vi "Parse Semver Range.vi"(8 "error in (no error)":errorcluster, 9 "Offset in":i32, 10 "Range Specifier":string) -> (0 "error out":errorcluster, 1 "Offset out":i32, 2 "Operator":string, 3 "Semver out":refnum<class "Semver.lvclass">)   [LabVIEW 2017, in "Semver.lvlib" / "Semver.lvclass"]
uses:
  Semver.lvclass
  Semver.lvclass/Semver.ctl
  <vilib>/Utility/error.llb/Error Cluster From Error Code.vi
  <vilib>/ErrorRing/Error Ring.xnode
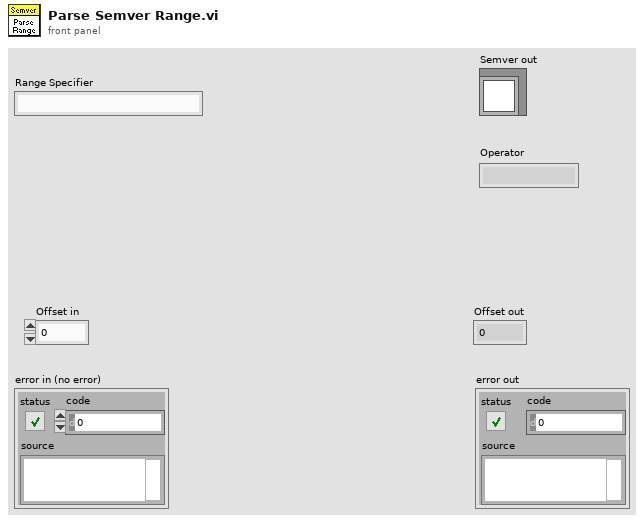
[diagram p1: front panel]
types:
  T1 = enum16{"Strip Chars", "Find Major", "Find Minor", "Find Patch", "Find Pre-Release", "Find Meta-Data"}
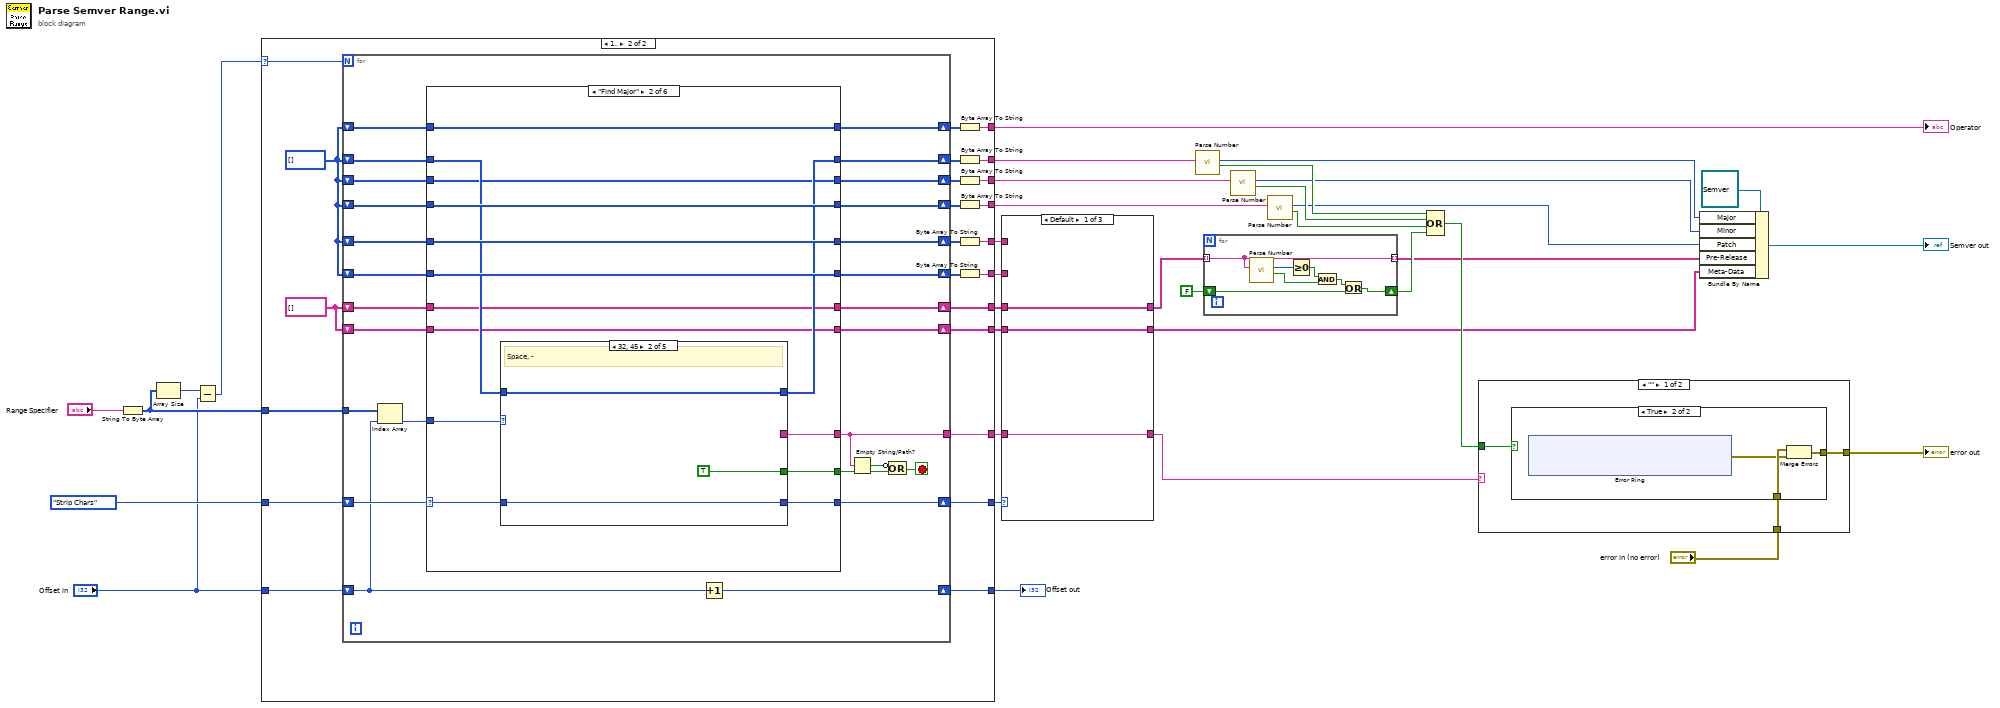
[diagram p0: block diagram]
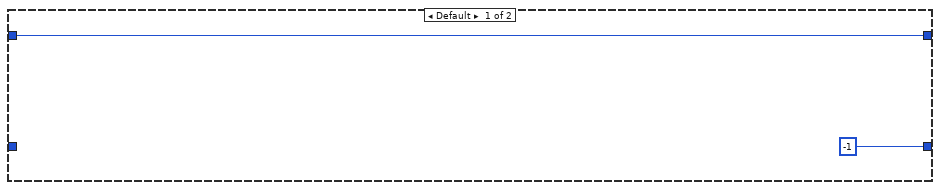
[diagram p2: hidden frame]
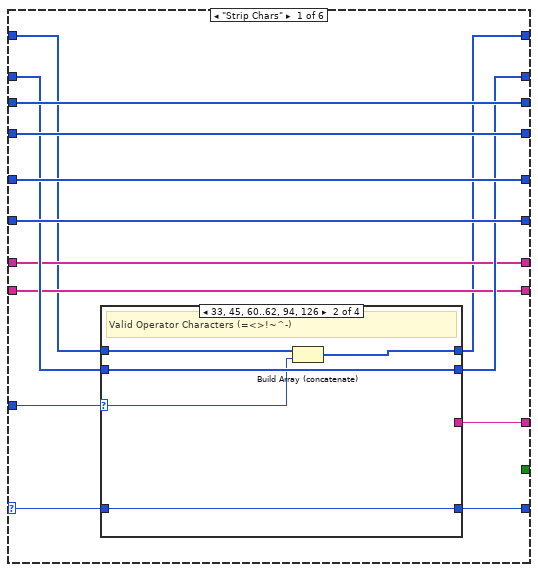
[diagram p3: hidden frame]
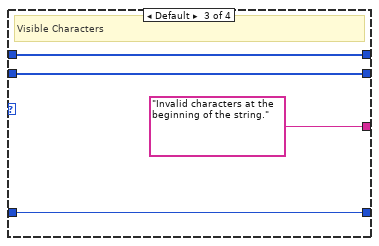
[diagram p5: hidden frame]
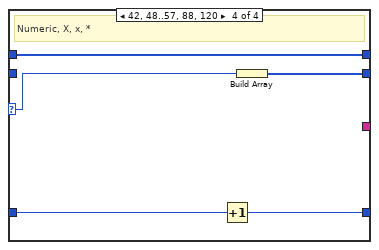
[diagram p6: hidden frame]
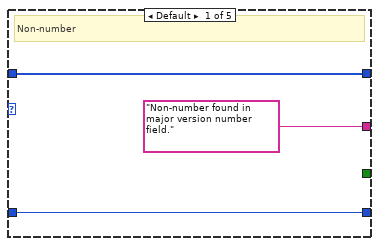
[diagram p7: hidden frame]
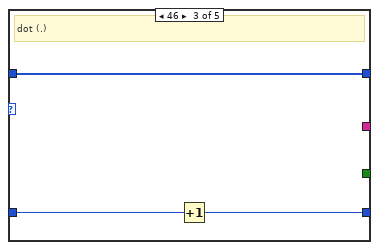
[diagram p8: hidden frame]
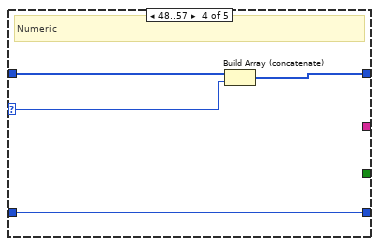
[diagram p9: hidden frame]
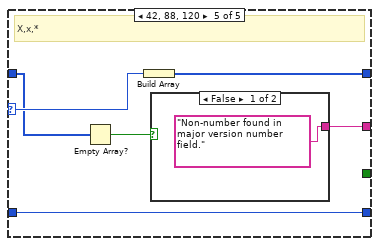
[diagram p10: hidden frame]
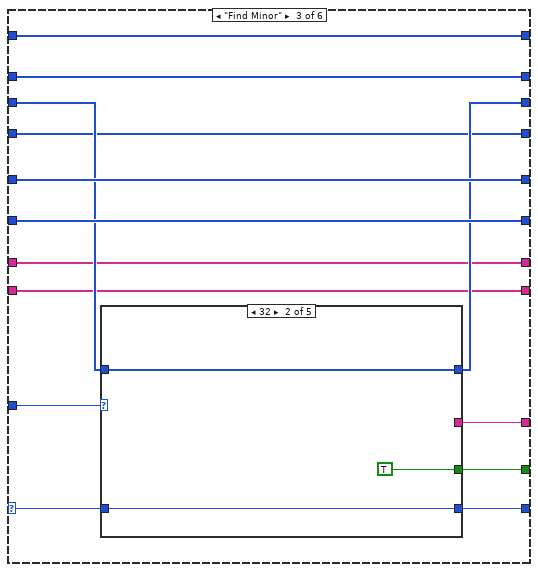
[diagram p12: hidden frame]
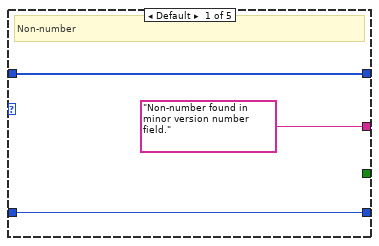
[diagram p13: hidden frame]
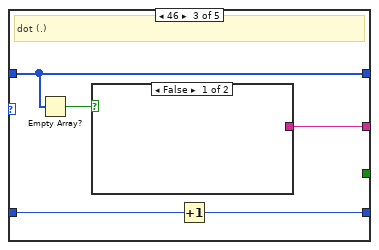
[diagram p14: hidden frame]
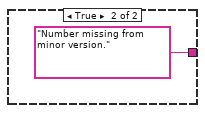
[diagram p15: hidden frame]
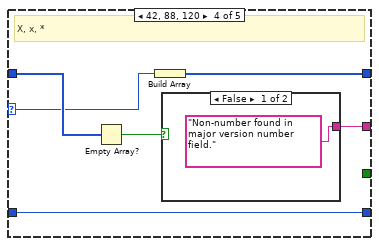
[diagram p16: hidden frame]
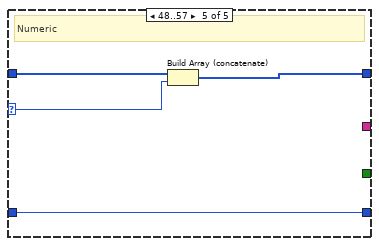
[diagram p18: hidden frame]
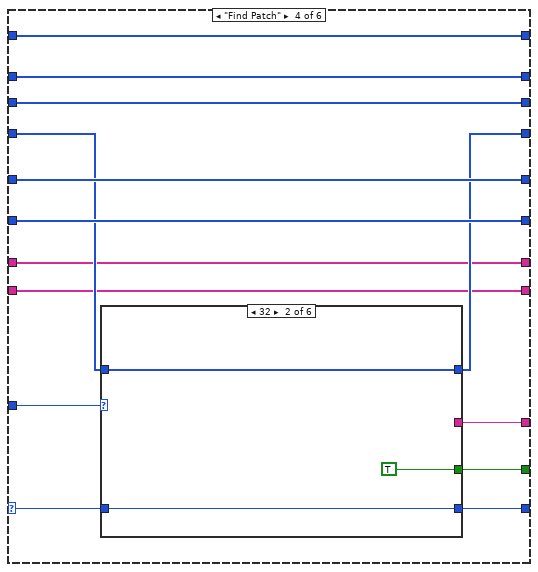
[diagram p19: hidden frame]
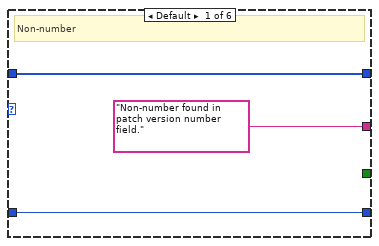
[diagram p20: hidden frame]
diagram:
  n1 = String To Byte Array(string="Range Specifier") -> (unsigned byte array=w4:u8[])
  n2 = Array Size(array=w4) -> (size(s)=w3:i32)
  n3 = Subtract(x=w3, y="Offset in") -> (x-y=w2:i32)
  n4 = case shown="1.." w2 {
    selector: w2 -> [_ w38]
    tunnel: T1."Strip Chars" -> [w36 w59]
    tunnel: [w36 w56] -> w32
    tunnel: [_ w55] -> w31
    tunnel: [_ w54] -> w30
    tunnel: [_ w53] -> w29
    tunnel: [_ w52] -> w28
    tunnel: [_ w51] -> w26
    tunnel: [_ w48] -> w23
    tunnel: [_ w47] -> w22
    tunnel: [_ w44] -> w21
    tunnel: [_ w41] -> w13
    tunnel: [-1 ("Offset in") w40] -> w5
    tunnel: w4 -> [_ w39]
    tunnel: "Offset in" -> [_ w37]
    frame Default {
    }
    frame 1.. {
      w50 = string[] []
      w42 = u8[] []
      n5 = for {
        N: w38 -> [_]
        tunnel: w39 -> [w66]
        shift-right: [w85] -> w49
        shift-left: w42 -> [w84]
        shift-right: [w83] -> w46
        shift-left: w42 -> [w82]
        shift-right: [w79] -> w45
        shift-left: w42 -> [w78]
        shift-right: [w80] -> w56
        shift-left: w59 -> [w81]
        shift-right: [w77] -> w57
        shift-left: w42 -> [w76]
        shift-right: [w74] -> w58
        shift-left: w42 -> [w75]
        shift-right: [w73] -> w54
        shift-left: w50 -> [w72]
        shift-right: [w70] -> w53
        shift-left: w50 -> [w71]
        tunnel: [w69] -> w51
        shift-right: [w67] -> w43
        shift-left: w42 -> [w68]
        shift-right: [w63] -> w40
        shift-left: w37 -> [w64]
        stop <- w60 stop-if-true
        n6 = Index Array(array=w66, index=w64) -> (element=w65:u8)
        n7 = case shown="\"Find Major\"" w81 {
          selector: w81 -> [w94 w126 w161 w198 w245 w283]
          tunnel: [w91 w123 w159 w196 w243 w281] -> w85
          tunnel: w84 -> [w92 w124 w159 w196 w243 w281]
          tunnel: [w99 w119 w157 w195 w242 w280] -> w83
          tunnel: w82 -> [w99 w119 w158 w195 w242 w280]
          tunnel: [w93 w125 w160 w197 w244 w282] -> w80
          tunnel: [w98 w130 w153 w193 w241 w279] -> w79
          tunnel: w78 -> [w98 w130 w153 w194 w241 w279]
          tunnel: [w97 w129 w164 w201 w238 w275] -> w77
          tunnel: w76 -> [w97 w129 w164 w201 w239 w275]
          tunnel: [w96 w128 w163 w200 w240 w276] -> w74
          tunnel: w75 -> [w96 w128 w163 w200 w240 w277]
          tunnel: w65 -> [w95 w127 w162 w199 w246 w284]
          tunnel: [w90 w122 w156 w192 w236 w278] -> w73
          tunnel: w72 -> [w90 w122 w156 w192 w237 w278]
          tunnel: w71 -> [w89 w121 w155 w191 w235 w274]
          tunnel: [w89 w121 w155 w191 w235 w273] -> w70
          tunnel: [w88 w120 w154 w190 w234 w272] -> w69
          tunnel: [w86 w118 w152 w189 w233 w271] -> w67
          tunnel: w68 -> [w87 w118 w152 w189 w233 w271]
          tunnel: [_ w117 w151 w188 w232 w270] -> w62
          frame "Strip Chars" {
            n8 = case shown="33, 45, 60..62, 94, 126" w95 {
              selector: w95 -> [_ w104 _ w114]
              tunnel: w94 -> [w102 w103 w111 w116]
              tunnel: [w102 w103 w111 w115] -> w93
              tunnel: w92 -> [w101 w107 w110 _]
              tunnel: [w101 w107 w110 w113] -> w91
              tunnel: [_ _ "Invalid characters at the beginning of the string." _] -> w88
              tunnel: [w100 w105 w108 w112] -> w86
              tunnel: w87 -> [w100 w106 w108 w112]
              frame 0..32, 118 {
                # "Whitespace, v"
              }
              frame 33, 45, 60..62, 94, 126 {
                # "Valid Operator Characters (=<>!~^-)"
                n9 = Build Array (concatenate)(w106, w104) -> (w105:u8[])
              }
              frame Default {
                # "Visible Characters"
              }
              frame 42, 48..57, 88, 120 {
                # "Numeric, X, x, *"
                n10 = Increment(x=w116) -> (x+1=w115:T1)
                n11 = Build Array(w114) -> (w113:u8[])
              }
            }
          }
          frame "Find Major" {
            n12 = case shown="32, 45" w127 {
              selector: w127 -> [_ _ _ w140 w149]
              tunnel: w126 -> [w133 w134 w139 w143 w144]
              tunnel: [w133 w134 w137 w143 w144] -> w125
              tunnel: w124 -> [w132 w136 w138 w142 w147]
              tunnel: [w132 w136 w138 w141 w148] -> w123
              tunnel: ["Non-number found in major version number field." _ _ _ w145] -> w120
              tunnel: [_ TRUE _ _ _] -> w117
              frame Default {
                # "Non-number"
              }
              frame 32, 45 {
                # "Space, -"
              }
              frame 46 {
                # "dot (.)"
                n13 = Increment(x=w139) -> (x+1=w137:T1)
              }
              frame 48..57 {
                # "Numeric"
                n14 = Build Array (concatenate)(w142, w140) -> (w141:u8[])
              }
              frame 42, 88, 120 {
                # "X,x,*"
                n15 = Empty Array?(array=w147) -> (empty?=w146:bool)
                n16 = Build Array(w149) -> (w148:u8[])
                n17 = case shown="False" w146 {
                  tunnel: ["Non-number found in major version number field." _] -> w145
                  frame False {
                  }
                  frame True {
                  }
                }
              }
            }
          }
          frame "Find Minor" {
            n18 = case shown="32" w162 {
              selector: w162 -> [_ _ _ w178 w184]
              tunnel: w161 -> [w167 w169 w175 w177 w187]
              tunnel: [w167 w169 w174 w177 w187] -> w160
              tunnel: w158 -> [w166 w170 w172 w181 w186]
              tunnel: [w166 w170 w172 w179 w185] -> w157
              tunnel: ["Non-number found in minor version number field." _ w173 w180 _] -> w154
              tunnel: [_ TRUE _ _ _] -> w151
              frame Default {
                # "Non-number"
              }
              frame 32 {
              }
              frame 46 {
                # "dot (.)"
                n19 = Empty Array?(array=w172) -> (empty?=w171:bool)
                n20 = case shown="False" w171 {
                  tunnel: [_ "Number missing from minor version."] -> w173
                  frame False {
                  }
                  frame True {
                  }
                }
                n21 = Increment(x=w175) -> (x+1=w174:T1)
              }
              frame 42, 88, 120 {
                # "X, x, *"
                n22 = Empty Array?(array=w181) -> (empty?=w182:bool)
                n23 = Build Array(w178) -> (w179:u8[])
                n24 = case shown="False" w182 {
                  tunnel: ["Non-number found in major version number field." _] -> w180
                  frame False {
                  }
                  frame True {
                  }
                }
              }
              frame 48..57 {
                # "Numeric"
                n25 = Build Array (concatenate)(w186, w184) -> (w185:u8[])
              }
            }
          }
          frame "Find Patch" {
            n26 = case shown="32" w199 {
              selector: w199 -> [_ _ _ _ w221 w228]
              tunnel: w198 -> [w204 w205 w212 w219 w224 w226]
              tunnel: [w204 w205 w211 w217 w224 w226] -> w197
              tunnel: w194 -> [w203 w207 w209 w215 w223 w229]
              tunnel: [w203 w207 w209 w215 w222 w225] -> w193
              tunnel: ["Non-number found in patch version number field." _ w210 w216 _ w227] -> w190
              tunnel: [_ TRUE _ _ _ _] -> w188
              frame Default {
                # "Non-number"
              }
              frame 32 {
              }
              frame 45 {
                # "hyphen (-)"
                n27 = Empty Array?(array=w209) -> (empty?=w208:bool)
                n28 = case shown="False" w208 {
                  tunnel: [_ "Patch number missing."] -> w210
                  frame False {
                  }
                  frame True {
                  }
                }
                n29 = Increment(x=w212) -> (x+1=w211:T1)
              }
              frame 43 {
                # "plus (+)"
                n30 = Empty Array?(array=w215) -> (empty?=w214:bool)
                n31 = case shown="False" w214 {
                  tunnel: [_ "Patch number missing."] -> w216
                  frame False {
                  }
                  frame True {
                  }
                }
                n32 = Increment(x=w219) -> (x+1=w218:T1)
                n33 = Increment(x=w218) -> (x+1=w217:T1)
              }
              frame 48..57 {
                # "Numeric"
                n34 = Build Array (concatenate)(w223, w221) -> (w222:u8[])
              }
              frame 42, 88, 120 {
                # "X, x *"
                n35 = Empty Array?(array=w229) -> (empty?=w230:bool)
                n36 = Build Array(w228) -> (w225:u8[])
                n37 = case shown="False" w230 {
                  tunnel: ["Non-number found in major version number field." _] -> w227
                  frame False {
                  }
                  frame True {
                  }
                }
              }
            }
          }
          frame "Find Pre-Release" {
            n38 = case shown="32" w246 {
              selector: w246 -> [_ _ _ _ w266]
              tunnel: w245 -> [w250 w251 w258 w260 w269]
              tunnel: [w250 w251 w257 w260 w269] -> w244
              tunnel: w239 -> [w249 w254 w256 w259 w268]
              tunnel: [w249 w254 w256 u8[] [] w267] -> w238
              tunnel: w237 -> [w248 w253 w255 w263 w265]
              tunnel: [w248 w253 w255 w262 w265] -> w236
              tunnel: ["Invalid character in pre-release identifier." _ _ _ _] -> w234
              tunnel: [_ TRUE _ _ _] -> w232
              frame Default {
                # "Invalid Char"
              }
              frame 32 {
              }
              frame 43 {
                # "plus (+)"
                n39 = Increment(x=w258) -> (x+1=w257:T1)
              }
              frame 46 {
                # "dot (.)"
                n40 = Byte Array To String(unsigned byte array=w259) -> (string=w261:string)
                n41 = Build Array (concatenate)(w263, w261) -> (w262:string[])
              }
              frame 48..57, 65..90, 97..122 {
                # "A-Za-z"
                n42 = Build Array (concatenate)(w268, w266) -> (w267:u8[])
              }
            }
          }
          frame "Find Meta-Data" {
            n43 = case shown="46" w284 {
              selector: w284 -> [_ _ w297 w301]
              tunnel: w283 -> [w288 w291 w300 w305]
              tunnel: [w288 w291 w300 w305] -> w282
              tunnel: w277 -> [w287 w290 w299 w302]
              tunnel: [w287 u8[] [] w298 w304] -> w276
              tunnel: w274 -> [w286 w294 w296 w303]
              tunnel: [w286 w293 w296 w303] -> w273
              tunnel: ["Invalid character in pre-release identifier." _ _ _] -> w272
              tunnel: [_ TRUE _ _] -> w270
              frame Default {
                # "Invalid Char"
              }
              frame 46 {
                # "dot (.)"
                n44 = Byte Array To String(unsigned byte array=w290) -> (string=w292:string)
                n45 = Build Array (concatenate)(w294, w292) -> (w293:string[])
              }
              frame 65..90, 97..122 {
                # "A-Za-z"
                n46 = Build Array (concatenate)(w299, w297) -> (w298:u8[])
              }
              frame 48..57 {
                # "A-Za-z"
                n47 = Build Array (concatenate)(w302, w301) -> (w304:u8[])
              }
            }
          }
        }
        n48 = Increment(x=w64) -> (x+1=w63:i32)
        n49 = Empty String/Path?(string/path=w69) -> (empty?=w61:bool)
        n50 = Compound Arithmetic op=OR(invert w61, w62) -> (w60:bool)
      }
      n51 = Byte Array To String(unsigned byte array=w43) -> (string=w41:string)
      n52 = Byte Array To String(unsigned byte array=w49) -> (string=w48:string)
      n53 = Byte Array To String(unsigned byte array=w46) -> (string=w47:string)
      n54 = Byte Array To String(unsigned byte array=w45) -> (string=w44:string)
      n55 = Byte Array To String(unsigned byte array=w57) -> (string=w55:string)
      n56 = Byte Array To String(unsigned byte array=w58) -> (string=w52:string)
    }
  }
  "Operator" <- w13
  "Offset out" <- w5
  n57 = case shown="Default" w32 {
    tunnel: w31 -> [_ w310 w317]
    tunnel: [w308 w311 w318] -> w17
    tunnel: w30 -> [w308 w313 w320]
    tunnel: [w307 w312 w316] -> w9
    tunnel: w29 -> [w307 w312 w319]
    tunnel: w28 -> [_ _ w315]
    tunnel: [w306 w309 w314] -> w27
    tunnel: w26 -> [w306 w309 w314]
    frame Default {
    }
    frame "Find Pre-Release" {
      n58 = Build Array (concatenate)(w313, w310) -> (w311:string[])
    }
    frame "Find Meta-Data" {
      n59 = Build Array (concatenate)(w319, w315) -> (w316:string[])
      n60 = Build Array (concatenate)(w320, w317) -> (w318:string[])
    }
  }
  n61 = call "Parse Number.vi"("String"=w23) -> ("Leading Zero?"=w20:bool, "Number"=w8:i32)  [unwired: 9 in]
  n62 = for {
    tunnel: [w327] -> w10 mode=indexing
    tunnel: w17 -> [w327] mode=indexing
    shift-right: [w322] -> w15
    shift-left: FALSE -> [w323]
    n63 = call "Parse Number.vi"("String"=w327) -> ("Leading Zero?"=w324:bool, "Number"=w326:i32)  [unwired: 9 in]
    n64 = Greater Or Equal To 0?(x=w326) -> (x >= 0?=w325:bool)
    n65 = And(x=w325, y=w324) -> (x .and. y?=w321:bool)
    n66 = Or(x=w321, y=w323) -> (x .or. y?=w322:bool)
  }
  n67 = call "Parse Number.vi"("String"=w22) -> ("Leading Zero?"=w19:bool, "Number"=w7:i32)  [unwired: 9 in]
  n68 = call "Parse Number.vi"("String"=w21) -> ("Leading Zero?"=w18:bool, "Number"=w6:i32)  [unwired: 9 in]
  n69 = Compound Arithmetic op=OR(w20, w19, w18, w15) -> (w14:bool)
  n70 = case shown="\"\"" w27 {
    selector: w27 -> [_ w343]
    tunnel: [w328 w340] -> w25
    tunnel: "error in (no error)" -> [w329 w341]
    tunnel: w14 -> [w330 _]
    frame "" {
      n71 = case shown="True" w330 {
        tunnel: w329 -> [w331 w333]
        tunnel: [w331 w334] -> w328
        frame False {
        }
        frame True {
          n72 = xnode "Error Ring"() -> ("error out"=w332:errorcluster)
          n73 = Merge Errors(w333, w332) -> (w334:errorcluster)
        }
      }
    }
    frame Default {
      n74 = xnode "Error Ring"("parameter 0"=w343) -> ("error out"=w342:errorcluster)
      n75 = Merge Errors(w341, w342) -> (w340:errorcluster)
    }
  }
  "error out" <- w25
  n76 = Bundle By Name(cluster=refnum<class "Semver.lvclass"> refnum ("Package Manager.lvlib:Semver.lvclass"), "Major"=w8, "Minor"=w7, "Patch"=w6, "Pre-Release"=w10, "Meta-Data"=w9) -> (→"Semver out":refnum<class "Semver.lvclass">)
